vi "Create Class Instance - Reentrant.vi"() -> (3 "SimpleArithmetic.lvclass":refnum<class "SimpleArithmetic - Reentrant.lvclass">)   [LabVIEW 2013]
uses:
  SimpleArithmetic - Reentrant.lvclass
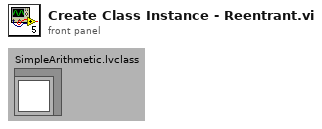
[diagram p1: front panel]
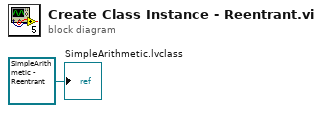
[diagram p0: block diagram]
diagram:
  "SimpleArithmetic.lvclass" <- refnum<class "SimpleArithmetic - Reentrant.lvclass"> refnum ("SimpleArithmetic.lvclass")
